vi "Write Sample.vi"(8 "error in (no error)":errorcluster, 9 "Sample":refnum<class "Sample.lvclass">, 10 "index":i32, 11 "Storage Line in":refnum<class "Storage Line.lvclass">) -> (0 "error out":errorcluster, 3 "Storage Line out":refnum<class "Storage Line.lvclass">)   [LabVIEW 2015, in "cRIO-Carbondioxide.lvlib" / "CO2-Actor.lvlib" / "Storage Line.lvclass"]
uses:
  Storage Line.lvclass
  subs/Sample/Sample.lvclass
  Storage Line.lvclass/Storage Line.ctl
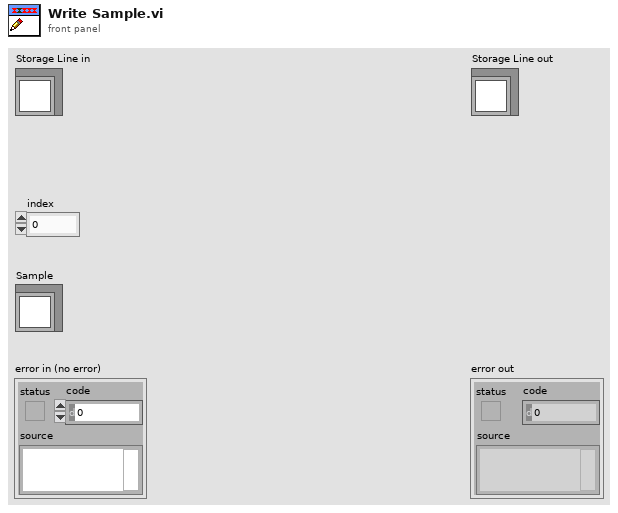
[diagram p1: front panel]
types:
  T1 = typedef "Sample Container.ctl" = cluster{"Sample In":refnum<k21>, "Sample Name":refnum<k21>, "Ti Cathode":refnum<k21>, "SampleQ":refnum<queue>}
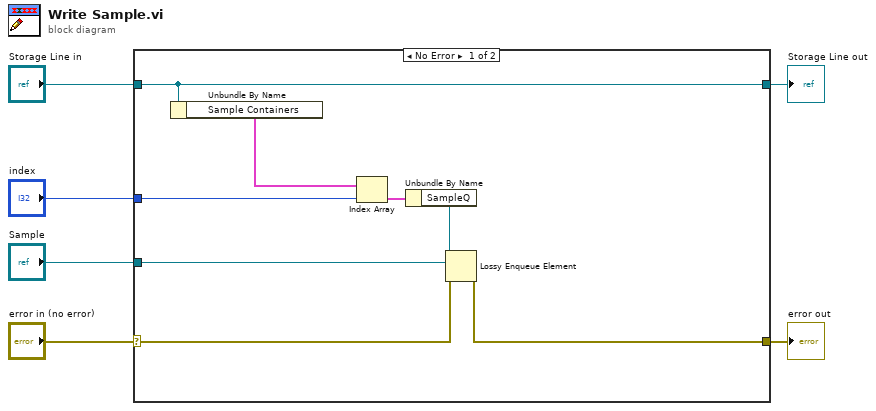
[diagram p0: block diagram]
diagram:
  n1 = case shown="No Error" "error in (no error)" {
    selector: "error in (no error)" -> [w8 w15]
    tunnel: [w7 w15] -> w5
    tunnel: [w14 w16] -> w3
    tunnel: "Storage Line in" -> [w14 w16]
    tunnel: "index" -> [w12 _]
    tunnel: "Sample" -> [w9 _]
    frame No Error {
      n2 = Unbundle By Name(w14) -> ("Sample Containers"=w13:T1[])
      n3 = Index Array(array=w13, index=w12) -> (element=w11:T1)
      n4 = Unbundle By Name(w11) -> ("SampleQ"=w10:refnum<queue>)
      n5 = Lossy Enqueue Element(queue=w10, element=w9, error in (no error)=w8) -> (error out=w7:errorcluster)  [unwired: 3 out]
    }
    frame Error {
    }
  }
  "error out" <- w5
  "Storage Line out" <- w3
